vi "Calibration-Frame11.vi"(0 "String in":refnum<vi>, 1 "reference in":refnum<vi>, 2 "Results file output":path, 3 "Array 5":dbl[](array[numeric]), 4 "Array 10":dbl[](array[numeric]), 6 "Array in":dbl[](array[numeric]), 7 "Array 6":dbl[](array[numeric]), 8 "data mode":enum16{"Take new data point", "Refit Curve"}(ring), 9 "Array 11":dbl[](array[numeric]), 11 "-ve Ref Values":bool) -> (10 "Array 8":dbl[](array[numeric]), 12 "Array 7":dbl[](array[numeric]), 13 "Status Out":T1, 14 "Array 9":dbl[](array[numeric]), 15 "Array 4":dbl[](array[numeric]), 16 "Array 3":dbl[](array[numeric]), 17 "String":string, 18 "Sample of input signals":dbl[][](graph))   [LabVIEW 2015]
uses:
  Anemometry Sub Vis/Gen Trav/Multi_Run_Status.ctl
  Anemometry Sub Vis/Controls/Setup.ctl
  Anemometry Sub Vis/Controls/Post_Process.ctl
  Anemometry Sub Vis/Controls/Save_Data.ctl
  <vilib>/Analysis/baseanly.llb/Mean (DBL).vi
  Anemometry Sub Vis/Globals/Calib_global.vi
  Anemometry Sub Vis/Globals/Meas_global.vi
  Anemometry Sub Vis/Acquisition/PWA/PWAtasksGLOBAL.vi
  <vilib>/Analysis/NI_AALBase.lvlib
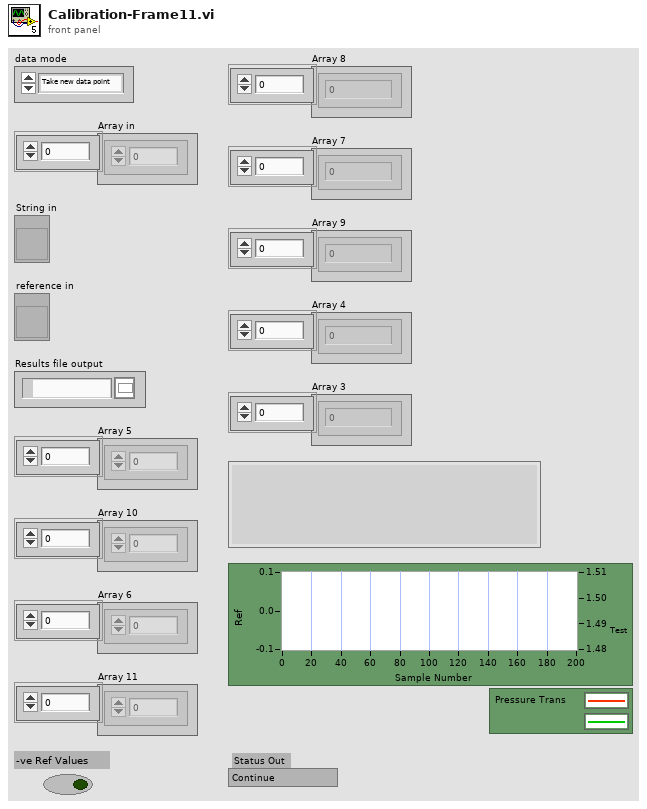
[diagram p1: front panel]
types:
  T1 = typedef "Multi_Run_Status.ctl" = enum16{"Continue", "Jump to Next Point", "Jump to Next Row", "Jump To Fall Back", "Terminate Run"}
  T2 = typedef "Ref_Inst_type.ctl" = enum16{"Propellor anemometer", "Pressure Transducer", "Raw voltage", "Pitot-static tube", "Preston tube", "Generic Linear", "Generic Polynomial", "Thermocouple", "LDA", "Enter Value", "ADAM Channel"}
  T3 = cluster{"2nd Ref type":T2, "2nd inst present":bool}
  T4 = typedef "Cal_Inst_type.ctl" = enum16{"Propeller anemometer", "Pressure Transducer", "Hot wire", "Cross wire velocity", "Cross wire angle", "Generic Linear", "Generic Polynomial", "Generic BackPoly", "Fast FID", "Thermocouple", "Cold wire", "Pulsed Wire"}
  T5 = typedef "Save_Data.ctl" = enum16{"Save No Data", "Save Data"}
  T6 = typedef "Post_Process.ctl" = enum16{"Take New Data", "Post Process Raw Data File"}
  T7 = typedef "Setup.ctl" = enum16{"Run Program", "Show Setup", "Save Current Setup", "Setup Front Panel"}
  T8 = typedef "Analysis_info_cluster.ctl" = cluster{"Colour":u32, "Inst type":T9, "Inst name":string, "Symbol":string, "Code name":string, "Extra Info":string, "Inst Array":T10, "Extra Titles":string[], "Extra Values":string[], "U":dbl, "u^2":dbl, "u^3":dbl, "u^4":dbl, "Skew_u":dbl, "Kurt_u":dbl, "Sd Error in Mean":dbl, "% u'/U":dbl, "X":dbl, "Y":dbl, "Z":dbl, "Timescale integral to 25%":dbl, "Sd Error in Variance":dbl, "Calib File":path, "Calib Constants":dbl[], "Output Position":bool, "Full Stats":bool, "Av Sampling Rate":dbl, "Av No of Samples":dbl, "Total Meas Time (s)":dbl, "ADAM Ch Name":string}
  T9 = typedef "Inst_type.ctl" = enum16{"Propeller anemometer", "Raw voltage", "Pressure Transducer", "Pitot-static tube", "Preston tube", "Hot wire", "Cross wire 1", "Cross wire 2", "Generic Linear", "Generic Polynomial", "Generic BackPoly", "Fast FID", "Thermocouple", "Cold wire", "Pulsed Wire", "LDA Vel", "LDA Tran time", "LDA Arr time", "Microphone"}
  T10 = typedef "Instrument_Array.ctl" = enum16{"PWA", "LDA", "Analogue"}
  T11 = typedef "Time_Trace_Cluster.ctl" = cluster{"Weighting":dbl[], "Time (s)":dbl[], "Voltage":dbl[], "Eng Values":dbl[]}
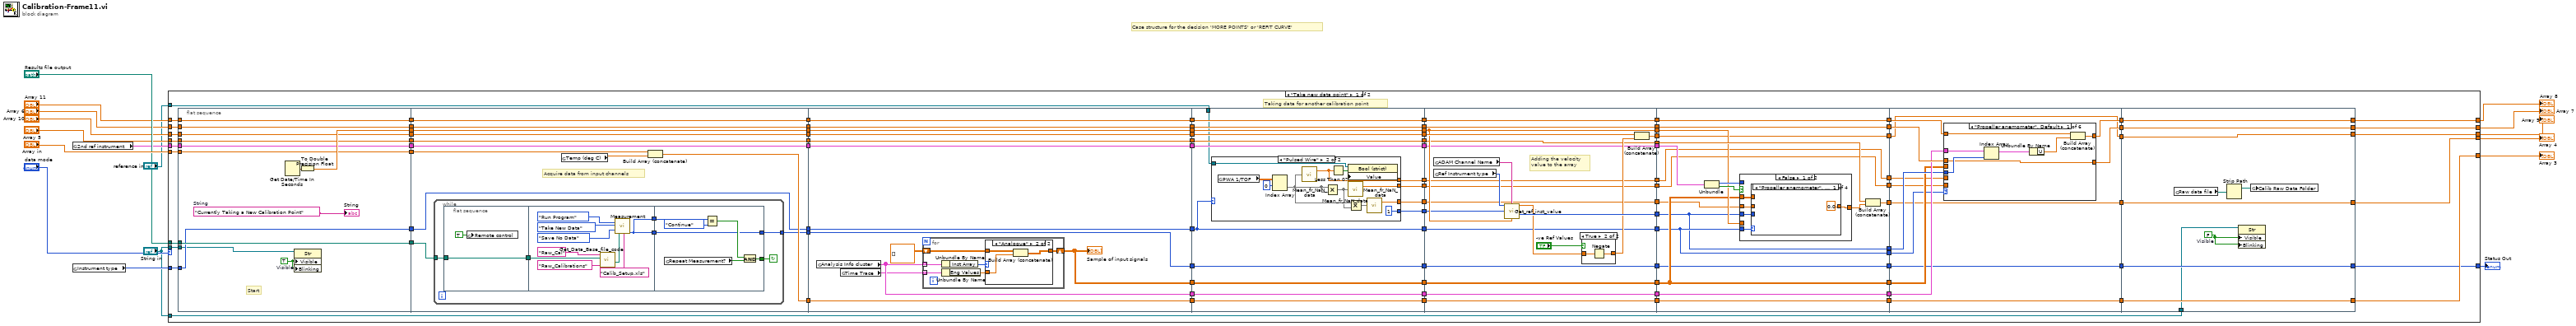
[diagram p0: block diagram]
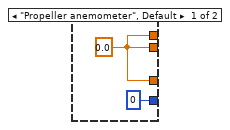
[diagram p3: hidden frame]
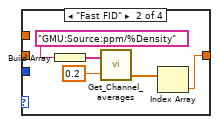
[diagram p5: hidden frame]
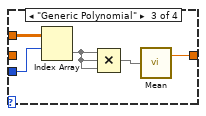
[diagram p6: hidden frame]
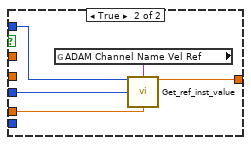
[diagram p8: hidden frame]
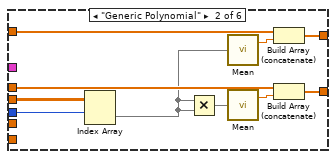
[diagram p9: hidden frame]
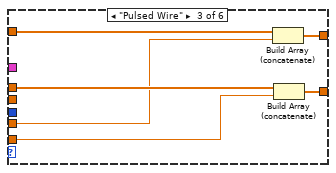
[diagram p10: hidden frame]
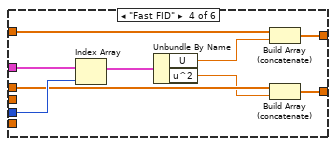
[diagram p11: hidden frame]
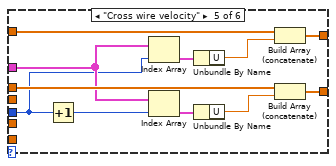
[diagram p12: hidden frame]
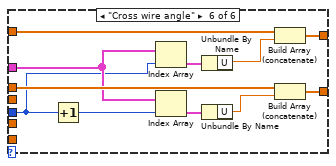
[diagram p13: hidden frame]
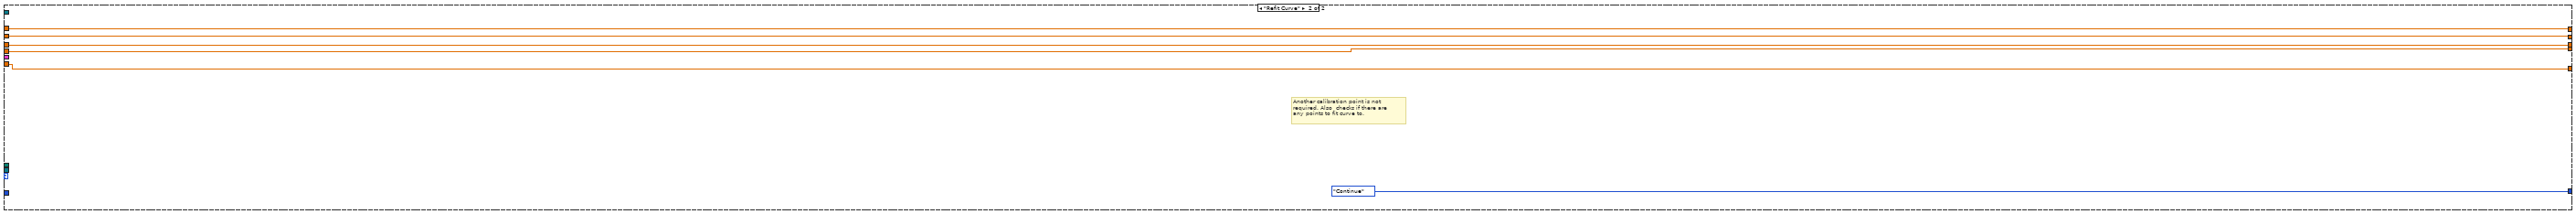
[diagram p14: hidden frame]
diagram:
  # "Case structure for the decision 'MORE POINTS' or 'REFIT CURVE'"
  n1 = global read "Calib_global.vi" "2nd ref instrument"() -> (w11:T3)
  n2 = global read "Calib_global.vi" "Instrument type"() -> (w16:T4)
  n3 = case shown="\"Take new data point\"" "data mode" {
    tunnel: [w108 w361] -> w6
    tunnel: [w109 w357] -> w5
    tunnel: "Array 11" -> [w110 w361]
    tunnel: "Array 10" -> [w111 w357]
    tunnel: [w107 w360] -> w7
    tunnel: "Array 6" -> [w106 w360]
    tunnel: "Array 5" -> [w105 w359]
    tunnel: [w103 w359] -> w10
    tunnel: w11 -> [w104 _]
    tunnel: [w101 w358] -> w12
    tunnel: "Array in" -> [w102 w358]
    tunnel: "Results file output" -> [w100 _]
    tunnel: [w99 Multi_Run_Status."Continue" ("Status Out")] -> w13
    tunnel: w16 -> [w98 _]
    tunnel: "String in" -> [w20 _]
    tunnel: "reference in" -> [w19 _]
    tunnel: "String in" -> [w18 _]
    frame "Take new data point" {
      # "Taking data for another calibration point"
      # "Start"
      n4 = flat-sequence {
        tunnel: w110 -> [w121]
        tunnel: [w121] -> w97
        tunnel: w111 -> [w120]
        tunnel: [w120] -> w96
        tunnel: w106 -> [w119]
        tunnel: [w119] -> w95
        tunnel: w105 -> [w118]
        tunnel: [w118] -> w94
        tunnel: w104 -> [w117]
        tunnel: [w117] -> w93
        tunnel: w102 -> [w116]
        tunnel: [w116] -> w92
        tunnel: w100 -> [w115]
        tunnel: [w115] -> w91
        tunnel: w98 -> [w114]
        tunnel: [w114] -> w90
        tunnel: [w124] -> w89
        tunnel: w20 -> [w112]
        tunnel: w97 -> [w131]
        tunnel: [w131] -> w88
        tunnel: w96 -> [w130]
        tunnel: [w130] -> w87
        tunnel: w95 -> [w129]
        tunnel: [w129] -> w86
        tunnel: w94 -> [w128]
        tunnel: [w128] -> w85
        tunnel: w93 -> [w127]
        tunnel: [w127] -> w84
        tunnel: w92 -> [w136]
        tunnel: [w135] -> w83
        tunnel: w91 -> [w133]
        tunnel: [w134] -> w82
        tunnel: w90 -> [w126]
        tunnel: [w126] -> w81
        tunnel: w89 -> [w125]
        tunnel: [w125] -> w80
        tunnel: w88 -> [w169]
        tunnel: [w169] -> w79
        tunnel: w87 -> [w168]
        tunnel: [w168] -> w78
        tunnel: w86 -> [w167]
        tunnel: [w167] -> w77
        tunnel: w85 -> [w166]
        tunnel: [w166] -> w76
        tunnel: w84 -> [w165]
        tunnel: [w165] -> w75
        tunnel: w83 -> [w164]
        tunnel: [w164] -> w74
        tunnel: w82 -> [w163]
        tunnel: [w163] -> w73
        tunnel: w81 -> [w162]
        tunnel: [w162] -> w72
        tunnel: w80 -> [w161]
        tunnel: [w161] -> w71
        tunnel: [w172] -> w70
        tunnel: [w160] -> w69
        tunnel: w79 -> [w194]
        tunnel: [w194] -> w68
        tunnel: w78 -> [w193]
        tunnel: [w193] -> w67
        tunnel: w77 -> [w192]
        tunnel: [w192] -> w66
        tunnel: w76 -> [w191]
        tunnel: [w191] -> w65
        tunnel: w75 -> [w190]
        tunnel: [w190] -> w64
        tunnel: w74 -> [w189]
        tunnel: [w189] -> w63
        tunnel: w73 -> [w188]
        tunnel: [w188] -> w62
        tunnel: w72 -> [w197]
        tunnel: [w197] -> w61
        tunnel: w71 -> [w187]
        tunnel: [w187] -> w60
        tunnel: w70 -> [w186]
        tunnel: [w186] -> w59
        tunnel: w69 -> [w185]
        tunnel: [w185] -> w58
        tunnel: [w198] -> w57
        tunnel: [w196] -> w56
        tunnel: [w195] -> w55
        tunnel: [w184] -> w54
        tunnel: w19 -> [w183]
        tunnel: w68 -> [w223]
        tunnel: [w223] -> w53
        tunnel: [w233] -> w52
        tunnel: w67 -> [w232]
        tunnel: w66 -> [w222]
        tunnel: [w222] -> w51
        tunnel: w65 -> [w221]
        tunnel: [w221] -> w50
        tunnel: w64 -> [w220]
        tunnel: [w220] -> w49
        tunnel: w63 -> [w219]
        tunnel: [w219] -> w48
        tunnel: w62 -> [w218]
        tunnel: [w218] -> w47
        tunnel: w61 -> [w217]
        tunnel: [w217] -> w46
        tunnel: [w230] -> w45
        tunnel: w60 -> [w231]
        tunnel: [w231] -> w44
        tunnel: w59 -> [w216]
        tunnel: [w216] -> w43
        tunnel: w58 -> [w215]
        tunnel: [w215] -> w42
        tunnel: w57 -> [w226]
        tunnel: w56 -> [w214]
        tunnel: [w214] -> w41
        tunnel: w55 -> [w213]
        tunnel: [w213] -> w40
        tunnel: w54 -> [w212]
        tunnel: [w212] -> w39
        tunnel: w53 -> [w245]
        tunnel: [w245] -> w38
        tunnel: w52 -> [w244]
        tunnel: [w244] -> w37
        tunnel: w51 -> [w243]
        tunnel: [w243] -> w36
        tunnel: w50 -> [w252]
        tunnel: [w251] -> w35
        tunnel: w49 -> [w250]
        tunnel: w48 -> [w242]
        tunnel: [w242] -> w34
        tunnel: w47 -> [w238]
        tunnel: [w238] -> w33
        tunnel: w46 -> [w247]
        tunnel: [w247] -> w32
        tunnel: w45 -> [w237]
        tunnel: w44 -> [w249]
        tunnel: w43 -> [w241]
        tunnel: [w241] -> w31
        tunnel: [w237] -> w30
        tunnel: w42 -> [w248]
        tunnel: [w248] -> w29
        tunnel: w41 -> [w240]
        tunnel: [w240] -> w28
        tunnel: w40 -> [w239]
        tunnel: [w239] -> w27
        tunnel: w39 -> [w246]
        tunnel: w38 -> [w291]
        tunnel: w37 -> [w281]
        tunnel: [w281] -> w26
        tunnel: [w290] -> w25
        tunnel: [w289] -> w24
        tunnel: w36 -> [w288]
        tunnel: w35 -> [w280]
        tunnel: [w280] -> w23
        tunnel: w34 -> [w279]
        tunnel: [w279] -> w22
        tunnel: w33 -> [w278]
        tunnel: [w278] -> w21
        tunnel: w32 -> [w284]
        tunnel: w31 -> [w287]
        tunnel: w30 -> [w286]
        tunnel: w29 -> [w285]
        tunnel: w28 -> [w283]
        tunnel: w27 -> [w282]
        tunnel: [w353] -> w109
        tunnel: w26 -> [w353]
        tunnel: [w352] -> w108
        tunnel: w25 -> [w352]
        tunnel: [w351] -> w107
        tunnel: w24 -> [w351]
        tunnel: [w350] -> w103
        tunnel: w23 -> [w350]
        tunnel: [w349] -> w101
        tunnel: w22 -> [w349]
        tunnel: [w348] -> w99
        tunnel: w21 -> [w348]
        tunnel: w18 -> [w346]
        frame #0 {
          w122 = TRUE  # Visible
          w113 = "Currently Taking a New Calibration Point"  # String
          n5 = Get Date/Time In Seconds() -> (seconds since 1Jan1904=w123:timestamp)
          n6 = property on="Property Node" class="Str"(reference=w112, "Visible"=w122, "Blinking"=w122) -> ()  [unwired: 1 in, 2 out]
          n7 = To Double Precision Float(number=w123) -> (double precision float=w124:dbl)
          "String" <- w113
        }
        frame #1 {
          # "Acquire data from input channels"
          n8 = while {
            tunnel: [w142] -> w134
            tunnel: w133 -> [w141]
            stop <- w140 continue-if-true
            n9 = flat-sequence {
              tunnel: w141 -> [w143]
              tunnel: [w143] -> w139
              tunnel: [w146] -> w138
              tunnel: w139 -> [w150]
              tunnel: [w146] -> w137
              tunnel: [w154] -> w142
              tunnel: w138 -> [w154]
              tunnel: [w156] -> w140
              tunnel: w137 -> [w155]
              frame #0 {
                n10 = global write "Meas_global.vi" "Remote control"(TRUE ("Remote control")) -> ()
              }
              frame #1 {
                n11 = call "Get_Data_Base_file_code.vi"("Data Type"="Raw_Calibrations", "Results Filename"=w150, "Short_Name"="Raw_Cal" ("Data Type")) -> ("Raw Data File Name"=w147:path)  [unwired: 1 in, 3 out]
                n12 = call "Measurement.vi"("setup"=Setup."Run Program", "Post Process"=Post_Process."Take New Data", "File"=Save_Data."Save No Data", "Raw data file"=w147, "Setup filename"="Calib_Setup.xls") -> ("Status Out"=w146:T1)  [unwired: 2 in, 12 out]
              }
              frame #2 {
                n13 = global read "Meas_global.vi" "Repeat Measurement?"() -> (w157:bool)
                n14 = Equal?(x=w155, y=Multi_Run_Status."Continue" ("Status Out")) -> (x = y?=w158:bool)
                n15 = And(x=w158, y=w157) -> (x .and. y?=w156:bool)
              }
            }
          }
          n16 = global read "Calib_global.vi" "Temp (deg C)"() -> (w132:dbl)
          n17 = Build Array (concatenate)(w136, w132) -> (w135:dbl[])
        }
        frame #2 {
          n18 = global read "Meas_global.vi" "Analysis Info cluster"() -> (w172:T8[])
          n19 = global read "Meas_global.vi" "Time Trace"() -> (w170:T11[])
          n20 = for {
            tunnel: w172 -> [w178] mode=indexing
            shift-right: [w175] -> w160
            shift-left: dbl[][] [] -> [w176]
            tunnel: w170 -> [w174] mode=indexing
            n21 = Unbundle By Name(w178) -> ("Inst Array"=w177:T10)
            n22 = Unbundle By Name(w174) -> ("Eng Values"=w173:dbl[])
            n23 = case shown="\"Analogue\"" w177 {
              tunnel: w176 -> [w179 w182]
              tunnel: w173 -> [_ w181]
              tunnel: [w179 w180] -> w175
              frame "PWA", Default {
              }
              frame "Analogue" {
                n24 = Build Array (concatenate)(w182, w181) -> (w180:dbl[][])
              }
            }
          }
          "Sample of input signals" <- w160
        }
        frame #3 {
          n25 = case shown="\"Pulsed Wire\"" w197 {
            tunnel: [0 ("Index in") 1 ("Index in")] -> w198
            tunnel: [w199 w203] -> w196
            tunnel: [w199 w207] -> w195
            tunnel: [w199 w206] -> w184
            tunnel: w183 -> [_ w201]
            frame "Propeller anemometer", Default {
              w199 = 0.0 ("mean")
            }
            frame "Pulsed Wire" {
              n26 = global read "PWAtasksGLOBAL.vi" "PWA 1/TOF"() -> (w210:dbl[][])
              n27 = Index Array(array=w210, index (row)=0) -> (element=w208:dbl[])  [unwired: 1 in]
              n28 = call "Mean_fr_NaN_data.vi"("Data"=w208) -> ("Mean value"=w203:dbl)  [unwired: 1 out]
              n29 = Multiply(x=w208, y=w208) -> (x*y=w205:dbl[])
              n30 = Less Than 0?(x=w203) -> (x < 0?=w202:bool)
              n31 = property class="Bool (strict)"(reference=w201, "Value"=w202) -> ()  [unwired: 1 in, 2 out]
              n32 = call "Mean_fr_NaN_data.vi"("Data"=w205) -> ("Mean value"=w207:dbl)  [unwired: 1 out]
              n33 = Multiply(x=w208, y=w205) -> (x*y=w204:dbl[])
              n34 = call "Mean_fr_NaN_data.vi"("Data"=w204) -> ("Mean value"=w206:dbl)  [unwired: 1 out]
            }
          }
        }
        frame #4 {
          # "Adding the velocity\nvalue to the array"
          n35 = global read "Calib_global.vi" "ADAM Channel Name"() -> (w224:string)
          n36 = global read "Calib_global.vi" "Ref Instrument type"() -> (w229:T2)
          n37 = call "Get_ref_inst_value.vi"("Ref Instrument type"=w229, "ADAM Channel Name"=w224, "Index in"=w226, "Start time"=w231) -> ("Ref Value"=w228:dbl, "Index out"=w230:i32)  [unwired: 3 in, 7 out]
          n38 = case shown="True" "-ve Ref Values" {
            tunnel: w228 -> [w234 w236]
            tunnel: [w234 w235] -> w227
            frame False {
            }
            frame True {
              n39 = Negate(x=w236) -> (-x=w235:dbl)
            }
          }
          n40 = Build Array (concatenate)(w232, w227) -> (w233:dbl[])
        }
        frame #5 {
          n41 = Unbundle(w250) -> ("2nd Ref type"=w254:T2, "2nd inst present"=w253:bool)
          n42 = case shown="False" w253 {
            tunnel: w237 -> [w260 w274]
            tunnel: [w258 w275] -> w255
            tunnel: w254 -> [_ w276]
            tunnel: w249 -> [_ w277]
            tunnel: w248 -> [w259 _]
            tunnel: w247 -> [w257 _]
            tunnel: w246 -> [w256 _]
            frame False {
              n43 = case shown="\"Propeller anemometer\", Default" w257 {
                tunnel: w260 -> [_ _ w271 _]
                tunnel: w259 -> [_ _ w270 _]
                tunnel: [0.0 ("mean") w262 w268 w272] -> w258
                tunnel: w256 -> [_ _ _ w272]
                frame "Propeller anemometer", Default {
                }
                frame "Fast FID" {
                  n44 = Build Array("GMU:Source:ppm/%Density") -> (w265:string[])
                  n45 = call "Get_Channel_averages.vi"("Desired Ch Names"=w265, "Averaging time (mins)"=0.2) -> ("number"=w263:dbl[])  [unwired: 1 in, 2 out]
                  n46 = Index Array(array=w263) -> (element=w262:dbl)  [unwired: 1 in]
                }
                frame "Generic Polynomial" {
                  n47 = Index Array(array=w270, index (row)=w271) -> (element=w267:dbl[])  [unwired: 1 in]
                  n48 = Compound Arithmetic op=MULTIPLY(w267, w267, w267) -> (w269:dbl[])
                  n49 = call-poly <vilib>:"Mean.vi"("X"=w269) -> ("mean"=w268:dbl)  [unwired: 1 out]
                }
                frame "Pulsed Wire" {
                }
              }
            }
            frame True {
              n50 = global read "Calib_global.vi" "ADAM Channel Name Vel Ref"() -> (w273:string)
              n51 = call "Get_ref_inst_value.vi"("Ref Instrument type"=w276, "ADAM Channel Name"=w273, "Index in"=w274, "Start time"=w277) -> ("Ref Value"=w275:dbl)  [unwired: 4 in, 7 out]
            }
          }
          n52 = Build Array (concatenate)(w252, w255) -> (w251:dbl[])
        }
        frame #6 {
          n53 = case shown="\"Propeller anemometer\", Default" w284 {
            tunnel: w291 -> [w296 w306 w313 w321 w333 w344]
            tunnel: [w297 w307 w314 w322 w334 w345] -> w290
            tunnel: w288 -> [w295 w305 w312 w317 w332 w343]
            tunnel: [w295 w304 w311 w315 w331 w342] -> w289
            tunnel: w287 -> [w293 _ _ w319 w327 w338]
            tunnel: w286 -> [w298 w308 _ w323 w325 w336]
            tunnel: w285 -> [_ w303 _ _ _ _]
            tunnel: w283 -> [_ _ w310 _ _ _]
            tunnel: w282 -> [_ _ w309 _ _ _]
            frame "Propeller anemometer", Default {
              n54 = Index Array(array=w293, index=w298) -> (element=w294:T8)
              n55 = Unbundle By Name(w294) -> ("U"=w292:dbl)
              n56 = Build Array (concatenate)(w296, w292) -> (w297:dbl[])
            }
            frame "Generic Polynomial" {
              n57 = Index Array(array=w303, index (row)=w308) -> (element=w300:dbl[])  [unwired: 1 in]
              n58 = Multiply(x=w300, y=w300) -> (x*y=w299:dbl[])
              n59 = call-poly <vilib>:"Mean.vi"("X"=w300) -> ("mean"=w302:dbl)  [unwired: 1 out]
              n60 = call-poly <vilib>:"Mean.vi"("X"=w299) -> ("mean"=w301:dbl)  [unwired: 1 out]
              n61 = Build Array (concatenate)(w306, w302) -> (w307:dbl[])
              n62 = Build Array (concatenate)(w305, w301) -> (w304:dbl[])
            }
            frame "Pulsed Wire" {
              n63 = Build Array (concatenate)(w313, w310) -> (w314:dbl[])
              n64 = Build Array (concatenate)(w312, w309) -> (w311:dbl[])
            }
            frame "Fast FID" {
              n65 = Index Array(array=w319, index=w323) -> (element=w320:T8)
              n66 = Unbundle By Name(w320) -> ("U"=w318:dbl, "u^2"=w316:dbl)
              n67 = Build Array (concatenate)(w321, w318) -> (w322:dbl[])
              n68 = Build Array (concatenate)(w317, w316) -> (w315:dbl[])
            }
            frame "Cross wire velocity" {
              n69 = Increment(x=w325) -> (x+1=w324:i32)
              n70 = Index Array(array=w327, index=w325) -> (element=w330:T8)
              n71 = Index Array(array=w327, index=w324) -> (element=w329:T8)
              n72 = Unbundle By Name(w330) -> ("U"=w326:dbl)
              n73 = Unbundle By Name(w329) -> ("U"=w328:dbl)
              n74 = Build Array (concatenate)(w333, w326) -> (w334:dbl[])
              n75 = Build Array (concatenate)(w332, w328) -> (w331:dbl[])
            }
            frame "Cross wire angle" {
              n76 = Increment(x=w336) -> (x+1=w335:i32)
              n77 = Index Array(array=w338, index=w336) -> (element=w341:T8)
              n78 = Index Array(array=w338, index=w335) -> (element=w340:T8)
              n79 = Unbundle By Name(w341) -> ("U"=w337:dbl)
              n80 = Unbundle By Name(w340) -> ("U"=w339:dbl)
              n81 = Build Array (concatenate)(w344, w337) -> (w345:dbl[])
              n82 = Build Array (concatenate)(w343, w339) -> (w342:dbl[])
            }
          }
        }
        frame #7 {
          w347 = FALSE  # Visible
          n83 = global read "Meas_global.vi" "Raw data file"() -> (w355:path)
          n84 = Strip Path(path=w355) -> (stripped path=w354:path)  [unwired: 1 out]
          n85 = property on="Property Node" class="Str"(reference=w346, "Visible"=w347, "Blinking"=w347) -> ()  [unwired: 1 in, 2 out]
          n86 = global write "Calib_global.vi" "Calib Raw Data Folder"(w354) -> ()
        }
      }
    }
    frame "Refit Curve" {
      # "Another calibration point is not\nrequired. Also  checks if there are\nany points to fit curve to."
    }
  }
  "Status Out" <- w13
  "Array 3" <- w12
  "Array 4" <- w10
  "Array 7" <- w7
  "Array 8" <- w6
  "Array 9" <- w5
